vi "dfd_Render ZPK Equation With Non-zero Delay.vi"(0 "picture in":picture, 1 "roots":cdb[](array[numeric]), 2 "gain":dbl=1.0, 3 "rect in":T3, 4 "alignment(left, top)":T2, 5 "delay":dbl, 6 "Fonts Input":T4(array[cluster]), 8 "format coeffiecients":string, 9 "bracket":cluster{"left":string, "right":string}={"left"="(", "right"=")"}, 10 "variable":string="z", 11 "display format":T1 items=["Separated Roots", "Combined Roots"]) -> (14 "picture out":picture, 17 "total rect":T3)   [LabVIEW 2017, in "NI_DigFilter_Process.lvlib"]
uses:
  <vilib>/addons/Digital Filter Design/NI_DigFilter_Process.lvlib
  <vilib>/addons/Digital Filter Design/Render.llb/dfd_ZPK Display Format.ctl
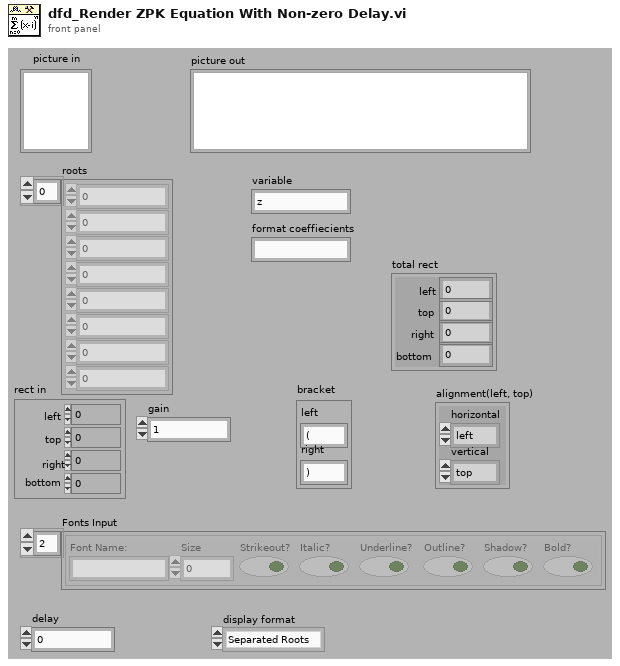
[diagram p1: front panel]
types:
  T1 = typedef "dfd_ZPK Display Format.ctl" = u16
  T2 = cluster{"horizontal":enum16{"left", "center", "right"}, "vertical":enum16{"top", "center", "bottom"}}
  T3 = cluster{"left":i16, "top":i16, "right":i16, "bottom":i16}
  T4 = cluster{"Font Name:":string, "Size":i16, "Strikeout?":bool, "Italic?":bool, "Underline?":bool, "Outline?":bool, "Shadow?":bool, "Bold?":bool}[]
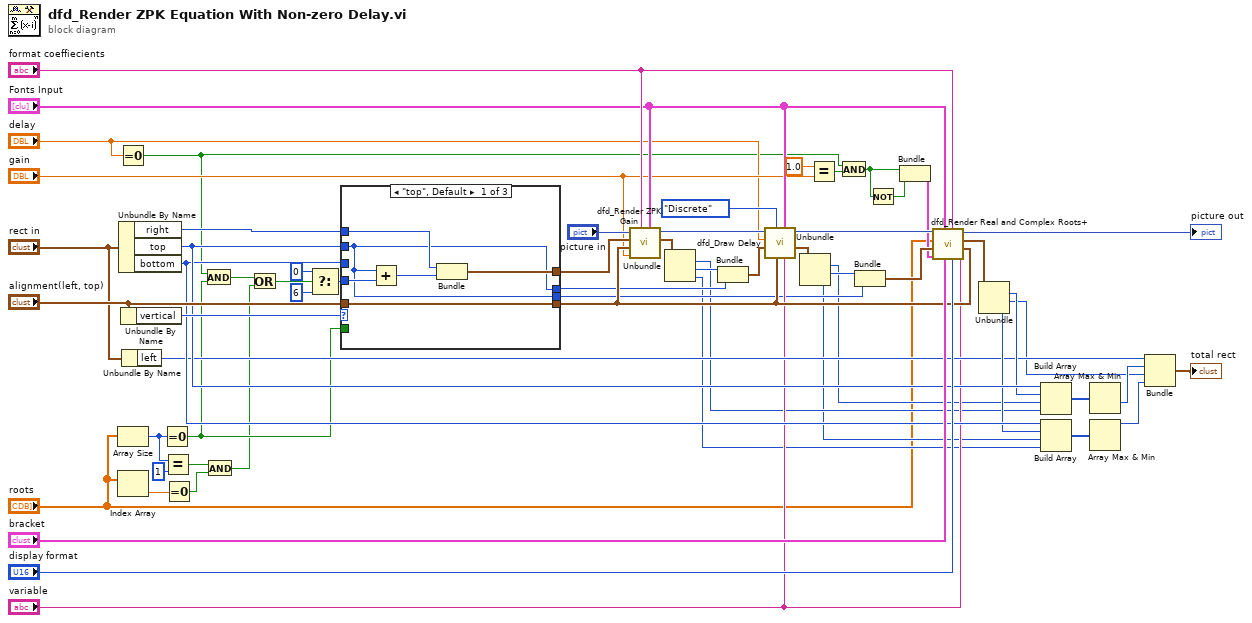
[diagram p0: block diagram]
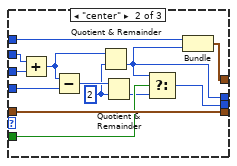
[diagram p2: hidden frame]
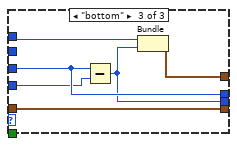
[diagram p3: hidden frame]
diagram:
  n1 = Equal To 0?(x="delay") -> (x = 0?=w14:bool)
  n2 = Array Size(array="roots") -> (size(s)=w7:i32)
  n3 = Index Array(array="roots") -> (element=w9:cdb)  [unwired: 1 in]
  n4 = Unbundle By Name("rect in") -> ("right"=w57:i16, "top"=w55:i16, "bottom"=w54:i16)
  n5 = Unbundle By Name("alignment(left, top)") -> ("vertical"=w61:enum16{"top", "center", "bottom"})
  n6 = Unbundle By Name("rect in") -> ("left"=w50:i16)
  n7 = Equal To 0?(x=w7) -> (x = 0?=w8:bool)
  n8 = Equal?(x=w7, y=1) -> (x = y?=w5:bool)
  n9 = Equal To 0?(x=w9) -> (x = 0?=w4:bool)
  n10 = And(x=w14, y=w8) -> (x .and. y?=w3:bool)
  n11 = And(x=w5, y=w4) -> (x .and. y?=w1:bool)
  n12 = Or(x=w3, y=w1) -> (x .or. y?=w2:bool)
  n13 = Select(t=0, s=w2, f=6) -> (s? t:f=w13:i32)
  n14 = case shown="\"top\", Default" w61 {
    tunnel: "alignment(left, top)" -> [w63 w74 w86]
    tunnel: [w63 w74 w86] -> w35
    tunnel: w57 -> [w65 w80 w85]
    tunnel: w55 -> [w62 w79 _]
    tunnel: w54 -> [_ w78 w83]
    tunnel: w13 -> [w67 w77 w82]
    tunnel: [w64 w72 w84] -> w43
    tunnel: [w62 w70 w83] -> w31
    tunnel: [w62 w68 w81] -> w29
    tunnel: w8 -> [_ w71 _]
    frame "top", Default {
      n15 = Add(x=w62, y=w67) -> (x+y=w66:i32)
      n16 = Bundle("right"=w65, w66) -> (w64:cluster{"right":i16, i32})  [unwired: 1 out]
    }
    frame "center" {
      w73 = i16 2 ("y")
      n17 = Add(x=w79, y=w78) -> (x+y=w75:i16)
      n18 = Subtract(x=w75, y=w77) -> (x-y=w76:i32)
      n19 = Quotient & Remainder(x=w75, y=w73) -> (floor(x/y)=w70:i16)  [unwired: 1 out]
      n20 = Quotient & Remainder(x=w76, y=w73) -> (floor(x/y)=w69:i32)  [unwired: 1 out]
      n21 = Select(t=w70, s=w71, f=w69) -> (s? t:f=w68:i32)
      n22 = Bundle("right"=w80, w70) -> (w72:cluster{"right":i16, i16})  [unwired: 1 out]
    }
    frame "bottom" {
      n23 = Subtract(x=w83, y=w82) -> (x-y=w81:i32)
      n24 = Bundle("right"=w85, w81) -> (w84:cluster{"right":i16, i32})  [unwired: 1 out]
    }
  }
  n25 = call <vilib>:"dfd_Render ZPK Gain.vi"("Fonts Input"="Fonts Input", "format coeffiecients"="format coeffiecients", "gain"="gain", "alignment(left, top)"=w35, "origin"=w43, "picture in"="picture in") -> ("text rect"=w38:T3, "picture out"=w42:picture)  [unwired: 2 in, 2 out]
  n26 = Unbundle(w38) -> ("top"=w25:i16, "right"=w37:i16, "bottom"=w24:i16)  [unwired: 1 out]
  n27 = Bundle("right"=w37, "bottom"=w31) -> (w36:cluster{"right":i16, "bottom":i16})  [unwired: 1 out]
  n28 = call <vilib>:"dfd_Draw Delay.vi"("variable"="variable", "fonts input"="Fonts Input", "alignment(left, top)"=w35, "equation type"=enum16{"Continuous", "Discrete"}."Discrete", "origin"=w36, "delay"="delay", "picture"=w42) -> ("text rect"=w34:T3, "new picture"=w41:picture)  [unwired: 3 out]
  n29 = Unbundle(w34) -> ("top"=w26:i16, "right"=w32:i16, "bottom"=w23:i16)  [unwired: 1 out]
  n30 = Equal?(x=1.0, y="gain") -> (x = y?=w19:bool)
  n31 = And(x=w14, y=w19) -> (x .and. y?=w17:bool)
  n32 = Bundle("right"=w32, "top"=w29) -> (w30:cluster{"right":i16, "top":i32})  [unwired: 1 out]
  n33 = Not(x=w17) -> (.not. x?=w16:bool)
  n34 = Bundle(w17, w16) -> (w15:cluster{bool, bool})  [unwired: 1 out]
  n35 = call <vilib>:"dfd_Render Real and Complex Roots+.vi"("variable"="variable", "alignment(left, top)"=w35, "display format"="display format", "format coeffiecients"="format coeffiecients", "bracket"="bracket", "fonts input"="Fonts Input", "format control"=w15, "origin"=w30, "Roots"="roots", "picture in"=w41) -> ("total rect"=w56:T3, "picture out"=→"picture out":picture)
  n36 = Unbundle(w56) -> ("top"=w53:i16, "right"=w22:i16, "bottom"=w52:i16)  [unwired: 1 out]
  n37 = Build Array(w55, w53, w26, w25) -> (w49:i16[])
  n38 = Build Array(w54, w52, w23, w24) -> (w47:i16[])
  n39 = Array Max & Min(array=w49) -> (min value=w48:i16)  [unwired: 3 out]
  n40 = Array Max & Min(array=w47) -> (max value=w46:i16)  [unwired: 3 out]
  n41 = Bundle("left"=w50, w48, "right"=w22, w46) -> (→"total rect":cluster{"left":i16, i16, "right":i16, i16})  [unwired: 1 out]
